vi "Ramp Actuator Speed.vi"(8 "error in (no error)":errorcluster, 9 "RA Down Volt":dbl, 10 "RA Up Volt":dbl, 11 "AIDeviceRef":T1) -> (2 "Ramp Actuator Ouput":dbl)   [LabVIEW 2011]
uses:
  <vilib>/Rock Robotics/WPI/AnalogChannel/WPI_AnalogChannelDevRef.ctl
  <vilib>/Rock Robotics/SystemInterfaces/Typedef/FPGA_TypedefAnalogModule.ctl
  <vilib>/Rock Robotics/SystemInterfaces/AI/FPGA_AIChannel.ctl
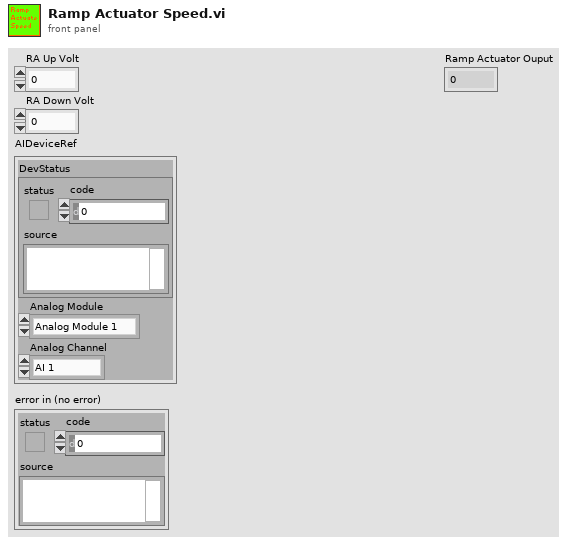
[diagram p1: front panel]
types:
  T1 = typedef "WPI_AnalogChannelDevRef.ctl" = cluster{"DevStatus":errorcluster, "Analog Module":T2, "Analog Channel":T3}
  T2 = typedef "FPGA_TypedefAnalogModule.ctl" = enum16{"Analog Module 1", "Analog Module 2"}
  T3 = typedef "FPGA_AIChannel.ctl" = enum8{"AI 1", "AI 2", "AI 3", "AI 4", "AI 5", "AI 6", "AI 7", "AI 8", "Invalid"}
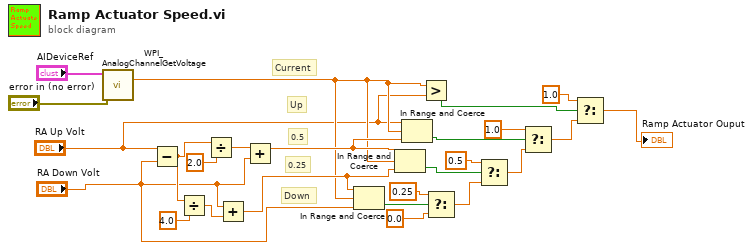
[diagram p0: block diagram]
diagram:
  # "Current"
  # "Down"
  # "0.25"
  # "0.5"
  # "Up"
  n1 = call <vilib>:"WPI_AnalogChannelGetVoltage.vi"("error in (no error)"="error in (no error)", "AIDeviceRef"="AIDeviceRef") -> ("Voltage"=w6:dbl)  [unwired: 7 in, 2 out]
  n2 = Subtract(x="RA Up Volt", y="RA Down Volt") -> (x-y=w22:dbl)
  n3 = Divide(x=w22, y=4.0) -> (x/y=w21:dbl)
  n4 = Divide(x=w22, y=2.0) -> (x/y=w23:dbl)
  n5 = Add(x="RA Down Volt", y=w21) -> (x+y=w11:dbl)
  n6 = Add(x=w23, y="RA Down Volt") -> (x+y=w10:dbl)
  n7 = In Range and Coerce(upper limit=w11, x=w6, lower limit="RA Down Volt") -> (In Range?=w13:bool)  [unwired: 1 out]
  n8 = In Range and Coerce(upper limit=w10, x=w6, lower limit=w11) -> (In Range?=w17:bool)  [unwired: 1 out]
  n9 = In Range and Coerce(upper limit="RA Up Volt", x=w6, lower limit=w10) -> (In Range?=w12:bool)  [unwired: 1 out]
  n10 = Greater?(x=w6, y="RA Up Volt") -> (0:w4:bool)
  n11 = Select(t=0.25, s=w13, f=0.0) -> (s? t:f=w16:dbl)
  n12 = Select(t=0.5, s=w17, f=w16) -> (s? t:f=w19:dbl)
  n13 = Select(t=1.0, s=w12, f=w19) -> (s? t:f=w2:dbl)
  n14 = Select(t=1.0, s=w4, f=w2) -> (s? t:f=→"Ramp Actuator Ouput":dbl)
